vi "Generate Simulation Data v2.vi"(8 "error in (no error)":errorcluster) -> (2 "Error Out":errorcluster)   [LabVIEW 2018]
uses:
  <vilib>/Utility/file.llb/Read Delimited Spreadsheet (DBL).vi
panel:
  out "Motr Current":dbl[](array[numeric])
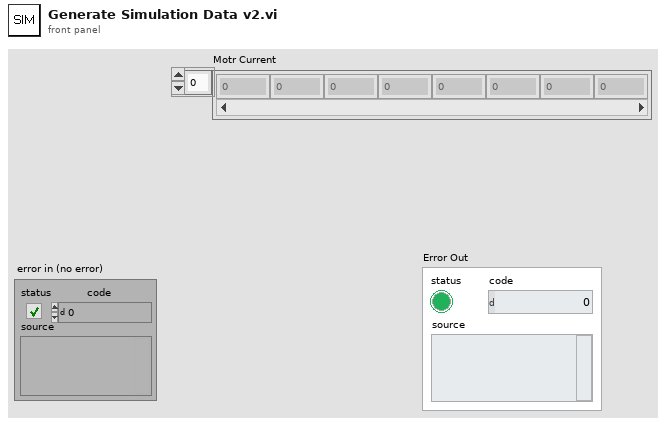
[diagram p1: front panel]
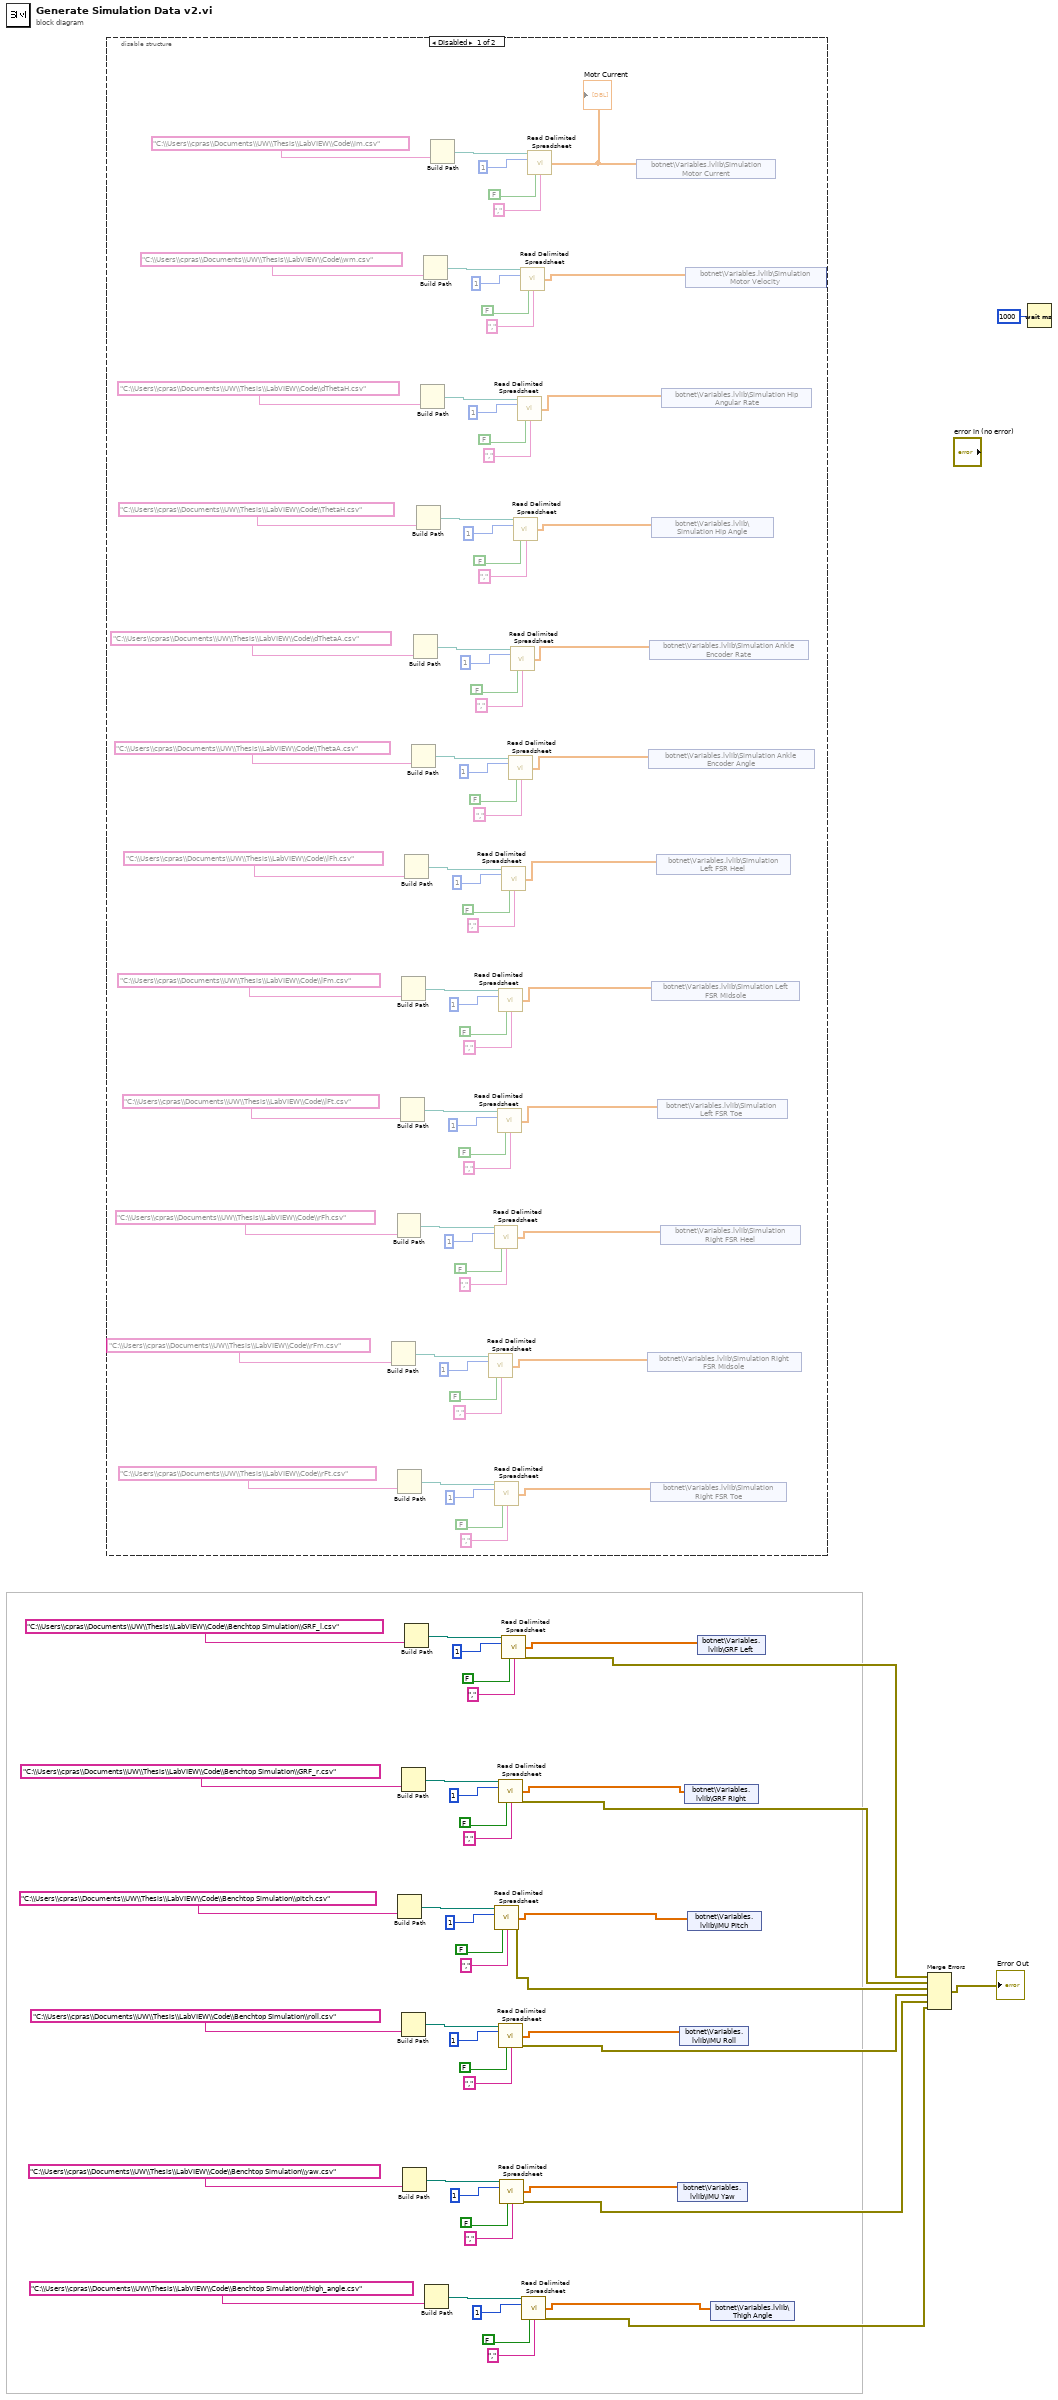
[diagram p0: block diagram]
diagram:
  n1 = disable-structure shown="Disabled" {
    frame Disabled {
      n2 = Build Path(name or relative path="C:\\Users\\cpras\\Documents\\UW\\Thesis\\LabVIEW\\Code\\rFm.csv") -> (appended path=w62:path)  [unwired: 1 in]
      n3 = Build Path(name or relative path="C:\\Users\\cpras\\Documents\\UW\\Thesis\\LabVIEW\\Code\\rFh.csv") -> (appended path=w71:path)  [unwired: 1 in]
      n4 = Build Path(name or relative path="C:\\Users\\cpras\\Documents\\UW\\Thesis\\LabVIEW\\Code\\rFt.csv") -> (appended path=w61:path)  [unwired: 1 in]
      n5 = Build Path(name or relative path="C:\\Users\\cpras\\Documents\\UW\\Thesis\\LabVIEW\\Code\\lFt.csv") -> (appended path=w72:path)  [unwired: 1 in]
      n6 = Build Path(name or relative path="C:\\Users\\cpras\\Documents\\UW\\Thesis\\LabVIEW\\Code\\lFm.csv") -> (appended path=w81:path)  [unwired: 1 in]
      n7 = Build Path(name or relative path="C:\\Users\\cpras\\Documents\\UW\\Thesis\\LabVIEW\\Code\\lFh.csv") -> (appended path=w82:path)  [unwired: 1 in]
      n8 = Build Path(name or relative path="C:\\Users\\cpras\\Documents\\UW\\Thesis\\LabVIEW\\Code\\ThetaA.csv") -> (appended path=w91:path)  [unwired: 1 in]
      n9 = Build Path(name or relative path="C:\\Users\\cpras\\Documents\\UW\\Thesis\\LabVIEW\\Code\\dThetaA.csv") -> (appended path=w92:path)  [unwired: 1 in]
      n10 = Build Path(name or relative path="C:\\Users\\cpras\\Documents\\UW\\Thesis\\LabVIEW\\Code\\ThetaH.csv") -> (appended path=w101:path)  [unwired: 1 in]
      n11 = Build Path(name or relative path="C:\\Users\\cpras\\Documents\\UW\\Thesis\\LabVIEW\\Code\\dThetaH.csv") -> (appended path=w102:path)  [unwired: 1 in]
      n12 = Build Path(name or relative path="C:\\Users\\cpras\\Documents\\UW\\Thesis\\LabVIEW\\Code\\wm.csv") -> (appended path=w111:path)  [unwired: 1 in]
      n13 = Build Path(name or relative path="C:\\Users\\cpras\\Documents\\UW\\Thesis\\LabVIEW\\Code\\im.csv") -> (appended path=w112:path)  [unwired: 1 in]
      n14 = call-poly <vilib>:"Read Delimited Spreadsheet.vi"("file path (dialog if empty)"=w62, "number of rows (all:-1)"=1, "transpose? (F)"=FALSE, "delimiter (\\t)"="," ("delimiter (\\t)")) -> ("first row"=w46:dbl[])  [unwired: 6 in, 5 out]
      n15 = call-poly <vilib>:"Read Delimited Spreadsheet.vi"("file path (dialog if empty)"=w71, "number of rows (all:-1)"=1, "transpose? (F)"=FALSE, "delimiter (\\t)"="," ("delimiter (\\t)")) -> ("first row"=w47:dbl[])  [unwired: 6 in, 5 out]
      n16 = call-poly <vilib>:"Read Delimited Spreadsheet.vi"("file path (dialog if empty)"=w61, "number of rows (all:-1)"=1, "transpose? (F)"=FALSE, "delimiter (\\t)"="," ("delimiter (\\t)")) -> ("first row"=w45:dbl[])  [unwired: 6 in, 5 out]
      n17 = call-poly <vilib>:"Read Delimited Spreadsheet.vi"("file path (dialog if empty)"=w72, "number of rows (all:-1)"=1, "transpose? (F)"=FALSE, "delimiter (\\t)"="," ("delimiter (\\t)")) -> ("first row"=w48:dbl[])  [unwired: 6 in, 5 out]
      n18 = call-poly <vilib>:"Read Delimited Spreadsheet.vi"("file path (dialog if empty)"=w81, "number of rows (all:-1)"=1, "transpose? (F)"=FALSE, "delimiter (\\t)"="," ("delimiter (\\t)")) -> ("first row"=w49:dbl[])  [unwired: 6 in, 5 out]
      n19 = call-poly <vilib>:"Read Delimited Spreadsheet.vi"("file path (dialog if empty)"=w82, "number of rows (all:-1)"=1, "transpose? (F)"=FALSE, "delimiter (\\t)"="," ("delimiter (\\t)")) -> ("first row"=w50:dbl[])  [unwired: 6 in, 5 out]
      n20 = call-poly <vilib>:"Read Delimited Spreadsheet.vi"("file path (dialog if empty)"=w91, "number of rows (all:-1)"=1, "transpose? (F)"=FALSE, "delimiter (\\t)"="," ("delimiter (\\t)")) -> ("first row"=w51:dbl[])  [unwired: 6 in, 5 out]
      n21 = call-poly <vilib>:"Read Delimited Spreadsheet.vi"("file path (dialog if empty)"=w92, "number of rows (all:-1)"=1, "transpose? (F)"=FALSE, "delimiter (\\t)"="," ("delimiter (\\t)")) -> ("first row"=w52:dbl[])  [unwired: 6 in, 5 out]
      n22 = call-poly <vilib>:"Read Delimited Spreadsheet.vi"("file path (dialog if empty)"=w101, "number of rows (all:-1)"=1, "transpose? (F)"=FALSE, "delimiter (\\t)"="," ("delimiter (\\t)")) -> ("first row"=w53:dbl[])  [unwired: 6 in, 5 out]
      n23 = call-poly <vilib>:"Read Delimited Spreadsheet.vi"("file path (dialog if empty)"=w102, "number of rows (all:-1)"=1, "transpose? (F)"=FALSE, "delimiter (\\t)"="," ("delimiter (\\t)")) -> ("first row"=w54:dbl[])  [unwired: 6 in, 5 out]
      n24 = call-poly <vilib>:"Read Delimited Spreadsheet.vi"("file path (dialog if empty)"=w111, "number of rows (all:-1)"=1, "transpose? (F)"=FALSE, "delimiter (\\t)"="," ("delimiter (\\t)")) -> ("first row"=w55:dbl[])  [unwired: 6 in, 5 out]
      n25 = call-poly <vilib>:"Read Delimited Spreadsheet.vi"("file path (dialog if empty)"=w112, "number of rows (all:-1)"=1, "transpose? (F)"=FALSE, "delimiter (\\t)"="," ("delimiter (\\t)")) -> ("first row"=w56:dbl[])  [unwired: 6 in, 5 out]
      "Motr Current" <- w56
      n26 = shared-variable "botnet\\Variables.lvlib\\Simulation Motor Current"(w56) -> ()  [unwired: 1 in, 1 out]
      n27 = shared-variable "botnet\\Variables.lvlib\\Simulation Right FSR Midsole"(w46) -> ()  [unwired: 1 in, 1 out]
      n28 = shared-variable "botnet\\Variables.lvlib\\Simulation Ankle Encoder Angle"(w51) -> ()  [unwired: 1 in, 1 out]
      n29 = shared-variable "botnet\\Variables.lvlib\\Simulation Ankle Encoder Rate"(w52) -> ()  [unwired: 1 in, 1 out]
      n30 = shared-variable "botnet\\Variables.lvlib\\Simulation Right FSR Toe"(w45) -> ()  [unwired: 1 in, 1 out]
      n31 = shared-variable "botnet\\Variables.lvlib\\Simulation Hip Angle"(w53) -> ()  [unwired: 1 in, 1 out]
      n32 = shared-variable "botnet\\Variables.lvlib\\Simulation Left FSR Midsole"(w49) -> ()  [unwired: 1 in, 1 out]
      n33 = shared-variable "botnet\\Variables.lvlib\\Simulation Left FSR Heel"(w50) -> ()  [unwired: 1 in, 1 out]
      n34 = shared-variable "botnet\\Variables.lvlib\\Simulation Left FSR Toe"(w48) -> ()  [unwired: 1 in, 1 out]
      n35 = shared-variable "botnet\\Variables.lvlib\\Simulation Right FSR Heel"(w47) -> ()  [unwired: 1 in, 1 out]
      n36 = shared-variable "botnet\\Variables.lvlib\\Simulation Hip Angular Rate"(w54) -> ()  [unwired: 1 in, 1 out]
      n37 = shared-variable "botnet\\Variables.lvlib\\Simulation Motor Velocity"(w55) -> ()  [unwired: 1 in, 1 out]
    }
    frame Enabled {
    }
  }
  n38 = Build Path(name or relative path="C:\\Users\\cpras\\Documents\\UW\\Thesis\\LabVIEW\\Code\\Benchtop Simulation\\pitch.csv") -> (appended path=w33:path)  [unwired: 1 in]
  n39 = Build Path(name or relative path="C:\\Users\\cpras\\Documents\\UW\\Thesis\\LabVIEW\\Code\\Benchtop Simulation\\GRF_r.csv") -> (appended path=w38:path)  [unwired: 1 in]
  n40 = Build Path(name or relative path="C:\\Users\\cpras\\Documents\\UW\\Thesis\\LabVIEW\\Code\\Benchtop Simulation\\roll.csv") -> (appended path=w28:path)  [unwired: 1 in]
  n41 = Build Path(name or relative path="C:\\Users\\cpras\\Documents\\UW\\Thesis\\LabVIEW\\Code\\Benchtop Simulation\\yaw.csv") -> (appended path=w23:path)  [unwired: 1 in]
  n42 = Build Path(name or relative path="C:\\Users\\cpras\\Documents\\UW\\Thesis\\LabVIEW\\Code\\Benchtop Simulation\\GRF_l.csv") -> (appended path=w43:path)  [unwired: 1 in]
  n43 = Build Path(name or relative path="C:\\Users\\cpras\\Documents\\UW\\Thesis\\LabVIEW\\Code\\Benchtop Simulation\\thigh_angle.csv") -> (appended path=w13:path)  [unwired: 1 in]
  n44 = call-poly <vilib>:"Read Delimited Spreadsheet.vi"("file path (dialog if empty)"=w33, "number of rows (all:-1)"=1, "transpose? (F)"=FALSE, "delimiter (\\t)"="," ("delimiter (\\t)")) -> ("first row"=w16:dbl[], "error out"=w5:errorcluster)  [unwired: 6 in, 4 out]
  n45 = call-poly <vilib>:"Read Delimited Spreadsheet.vi"("file path (dialog if empty)"=w38, "number of rows (all:-1)"=1, "transpose? (F)"=FALSE, "delimiter (\\t)"="," ("delimiter (\\t)")) -> ("first row"=w17:dbl[], "error out"=w6:errorcluster)  [unwired: 6 in, 4 out]
  n46 = call-poly <vilib>:"Read Delimited Spreadsheet.vi"("file path (dialog if empty)"=w28, "number of rows (all:-1)"=1, "transpose? (F)"=FALSE, "delimiter (\\t)"="," ("delimiter (\\t)")) -> ("first row"=w15:dbl[], "error out"=w4:errorcluster)  [unwired: 6 in, 4 out]
  n47 = call-poly <vilib>:"Read Delimited Spreadsheet.vi"("file path (dialog if empty)"=w23, "number of rows (all:-1)"=1, "transpose? (F)"=FALSE, "delimiter (\\t)"="," ("delimiter (\\t)")) -> ("first row"=w14:dbl[], "error out"=w3:errorcluster)  [unwired: 6 in, 4 out]
  n48 = call-poly <vilib>:"Read Delimited Spreadsheet.vi"("file path (dialog if empty)"=w43, "number of rows (all:-1)"=1, "transpose? (F)"=FALSE, "delimiter (\\t)"="," ("delimiter (\\t)")) -> ("first row"=w18:dbl[], "error out"=w7:errorcluster)  [unwired: 6 in, 4 out]
  n49 = call-poly <vilib>:"Read Delimited Spreadsheet.vi"("file path (dialog if empty)"=w13, "number of rows (all:-1)"=1, "transpose? (F)"=FALSE, "delimiter (\\t)"="," ("delimiter (\\t)")) -> ("first row"=w8:dbl[], "error out"=w2:errorcluster)  [unwired: 6 in, 4 out]
  n50 = shared-variable "botnet\\Variables.lvlib\\IMU Yaw"(w14) -> ()  [unwired: 1 in, 1 out]
  n51 = shared-variable "botnet\\Variables.lvlib\\IMU Roll"(w15) -> ()  [unwired: 1 in, 1 out]
  n52 = shared-variable "botnet\\Variables.lvlib\\GRF Right"(w17) -> ()  [unwired: 1 in, 1 out]
  n53 = shared-variable "botnet\\Variables.lvlib\\IMU Pitch"(w16) -> ()  [unwired: 1 in, 1 out]
  n54 = shared-variable "botnet\\Variables.lvlib\\GRF Left"(w18) -> ()  [unwired: 1 in, 1 out]
  n55 = shared-variable "botnet\\Variables.lvlib\\Thigh Angle"(w8) -> ()  [unwired: 1 in, 1 out]
  n56 = Merge Errors(w7, w6, w5, w4, w3, w2) -> (→"Error Out":errorcluster)
  n57 = Wait (ms)(milliseconds to wait=u32 1000) -> ()  [unwired: 1 out]
